vi "Configure Trigger (Pattern).vi"(0 "VISA resource name":refnum<visa-resource-name>, 1 "Analog Channel Pattern":string, 2 "Digital Channel Pattern":string, 5 "Pattern Condition (0:Entered)":u16(ring) items=["Entered", "Exited", "Greater Than", "Less Than", "Range"], 7 "Minimum Time (20e-9s)":dbl=2e-08, 9 "Maximum Time (50e-9s)":dbl=5e-08, 11 "error in (no error)":errorcluster) -> (4 "VISA resource name out":refnum<visa-resource-name>, 15 "error out":errorcluster)   [LabVIEW 2012, in "Agilent 8000 Series.lvlib"]
doc: "Configures the pattern trigger. It configures logic pattern to look for, the condition to trigger on, and the time limits for triggering."
uses:
  Agilent 8000 Series.lvlib
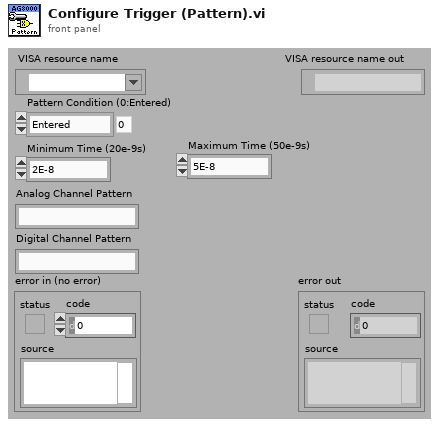
[diagram p1: front panel]
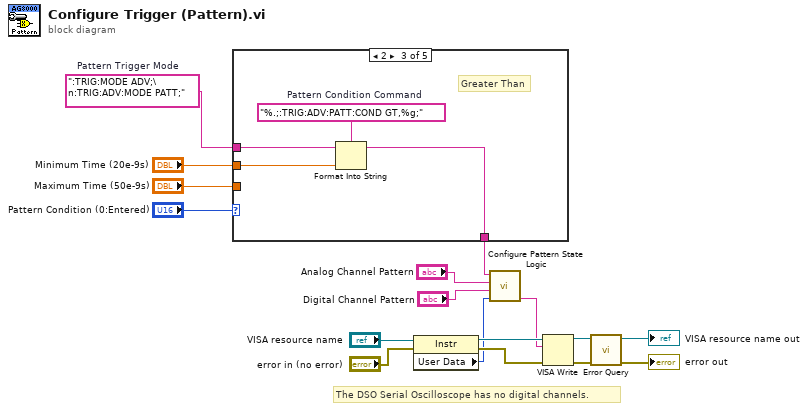
[diagram p0: block diagram]
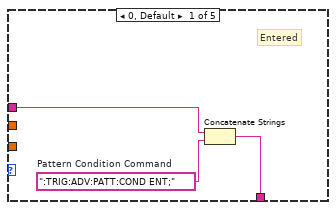
[diagram p2: hidden frame]
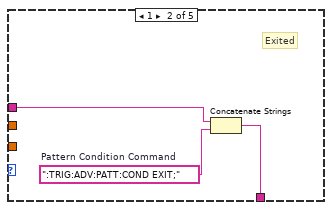
[diagram p3: hidden frame]
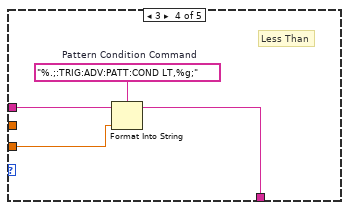
[diagram p4: hidden frame]
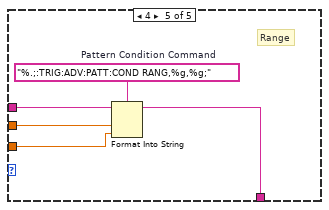
[diagram p5: hidden frame]
diagram:
  w10 = ":TRIG:MODE ADV;\n:TRIG:ADV:MODE PATT;"  # Pattern Trigger Mode
  # "The DSO Serial Oscilloscope has no digital channels."
  n1 = case shown="2" "Pattern Condition (0:Entered)" {
    tunnel: "Minimum Time (20e-9s)" -> [_ _ w26 _ w35]
    tunnel: "Maximum Time (50e-9s)" -> [_ _ _ w29 w34]
    tunnel: w10 -> [w20 w23 w25 w30 w33]
    tunnel: [w18 w21 w24 w28 w32] -> w9
    frame 0, Default {
      w19 = ":TRIG:ADV:PATT:COND ENT;"  # Pattern Condition Command
      # "Entered"
      n2 = Concatenate Strings(w20, w19) -> (w18:string)
    }
    frame 1 {
      w22 = ":TRIG:ADV:PATT:COND EXIT;"  # Pattern Condition Command
      # "Exited"
      n3 = Concatenate Strings(w23, w22) -> (w21:string)
    }
    frame 2 {
      w27 = "%.;:TRIG:ADV:PATT:COND GT,%g;"  # Pattern Condition Command
      # "Greater Than"
      n4 = Format Into String(format string=w27, initial string=w25, w26) -> (resulting string=w24:string)  [unwired: 1 in, 1 out]
    }
    frame 3 {
      w31 = "%.;:TRIG:ADV:PATT:COND LT,%g;"  # Pattern Condition Command
      # "Less Than"
      n5 = Format Into String(format string=w31, initial string=w30, w29) -> (resulting string=w28:string)  [unwired: 1 in, 1 out]
    }
    frame 4 {
      w36 = "%.;:TRIG:ADV:PATT:COND RANG,%g,%g;"  # Pattern Condition Command
      # "Range"
      n6 = Format Into String(format string=w36, initial string=w33, w35, w34) -> (resulting string=w32:string)  [unwired: 1 in, 1 out]
    }
  }
  n7 = property class="Instr"(reference="VISA resource name", error in="error in (no error)") -> (reference out=w7:refnum<visa-resource-name>, error out=w6:errorcluster, "User Data"=w3:u32)
  n8 = call "Configure Pattern State Logic.vi"("Model"=w3, "Digital Channel Pattern"="Digital Channel Pattern", "Analog Channel Pattern"="Analog Channel Pattern", "Input"=w9) -> ("Output"=w1:string)  [unwired: 7 in]
  n9 = VISA Write(VISA resource name=w7, write buffer=w1, error in (no error)=w6) -> (VISA resource name out=w15:refnum<visa-resource-name>, error out=w14:errorcluster)  [unwired: 1 out]
  n10 = call "Error Query.vi"("error in (no error)"=w14, "VISA resource name"=w15) -> ("error out"=→"error out":errorcluster, "VISA resource name out"=→"VISA resource name out":refnum<visa-resource-name>)  [unwired: 6 in, 2 out]
